vi "Get Version.vi"(8 "error in (no error)":errorcluster, 11 "Driver in":refnum<class "Driver.lvclass">) -> (0 "error out":errorcluster, 2 "Version":string, 3 "Driver out":refnum<class "Driver.lvclass">)   [LabVIEW 2023, in "Driver.lvlib" / "Driver.lvclass"]
uses:
  Driver.lvclass
  Driver.lvclass/Driver.ctl
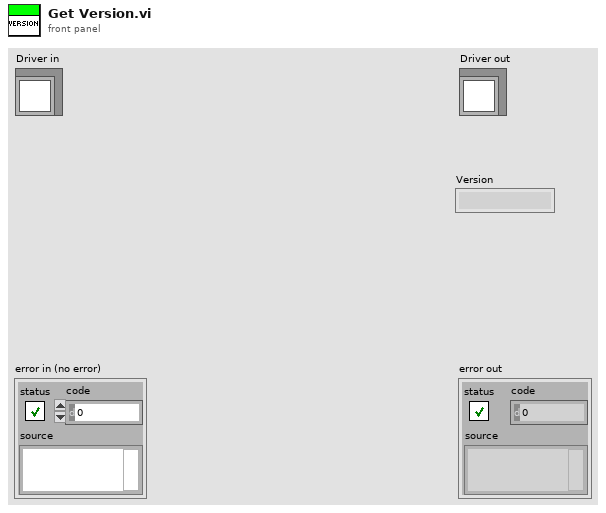
[diagram p1: front panel]
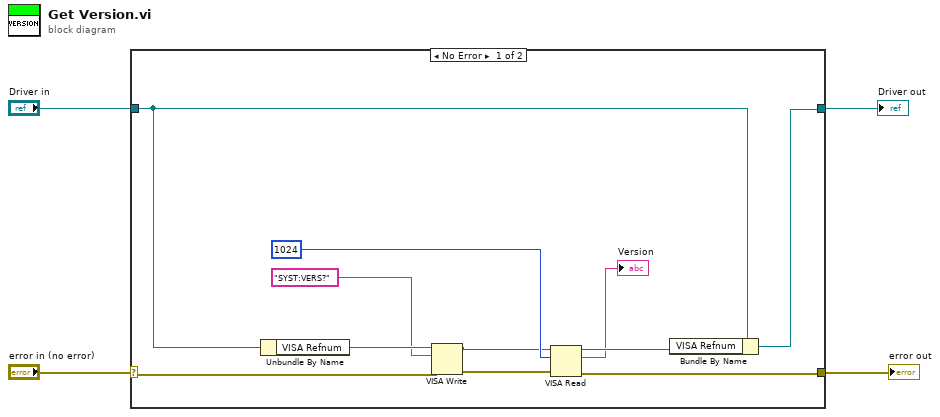
[diagram p0: block diagram]
diagram:
  n1 = case shown="No Error" "error in (no error)" {
    selector: "error in (no error)" -> [w10 w17]
    tunnel: [w9 w17] -> w3
    tunnel: [w7 w16] -> w1
    tunnel: "Driver in" -> [w8 w16]
    frame No Error {
      n2 = Unbundle By Name(w8) -> ("VISA Refnum"=w15:refnum<visa-resource-name>)
      n3 = VISA Write(VISA resource name=w15, write buffer="SYST:VERS?", error in (no error)=w10) -> (VISA resource name out=w11:refnum<visa-resource-name>, error out=w12:errorcluster)  [unwired: 1 out]
      n4 = VISA Read(VISA resource name=w11, byte count=u32 1024, error in (no error)=w12) -> (VISA resource name out=w6:refnum<visa-resource-name>, read buffer=→"Version":string, error out=w9:errorcluster)  [unwired: 1 out]
      n5 = Bundle By Name(cluster=w8, "VISA Refnum"=w6) -> (w7:refnum<class "Driver.lvclass">)
    }
    frame Error {
    }
  }
  "error out" <- w3
  "Driver out" <- w1
